vi "Read Connection Configuration.vi"(8 "error in (no error)":errorcluster, 11 "OPC UA configuration in":refnum<class "OPC UA Server configuration.lvclass">) -> (0 "error out":errorcluster, 2 "Connection Configuration":T2={"Client?"=FALSE, "Server Certificates"={"Relative Path?"=FALSE, "Certificate Paths"=[], "Certificate Names"=[]}, "Client Certificates"={"Relative Path?"=FALSE, "Certificate Paths"=[], "Certificate Names"=[]}, "Client Configuration"={"Server Endpoint URL"="", "Security Policy"={"Message Mode"=enum."None", "Security"=enum."Basic256"}, "Username/Password"={"Username"="", "Password"=""}}, "Server Configuration"={"Server Name"="", "TCP port (49580)"="49580", "Supported Security Policies"={"None"=TRUE, "Sign with Basic128Rsa125"=FALSE, "Sign and Encrypt with Basic128Rsa125"=FALSE, "Sign with Basic256"=FALSE, "Sign and Encrypt with Basic256"=FALSE}}}, 3 "OPC UA configuration out":refnum<class "OPC UA Server configuration.lvclass">)   [LabVIEW 2013, in "OPC UA Server configuration.lvclass"]
uses:
  OPC UA Server configuration.lvclass
  <vilib>/OPCUA/server/subVI/supported security policies.ctl
  OPC UA Server configuration.lvclass/OPC UA Server configuration.ctl
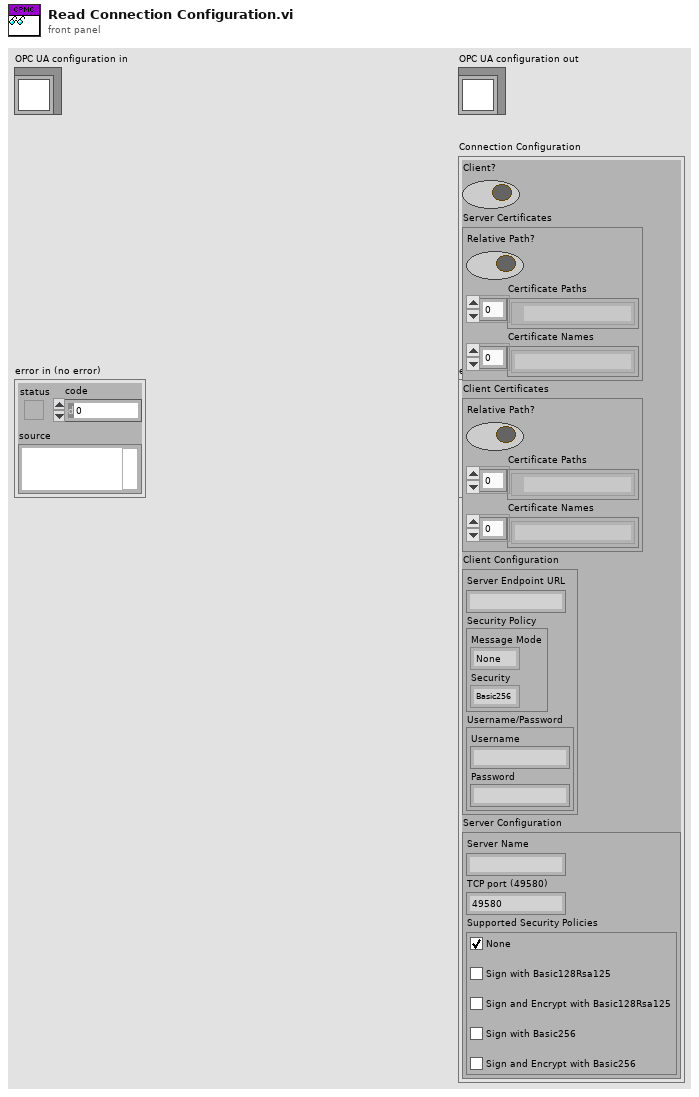
[diagram p1: front panel]
types:
  T1 = typedef "supported security policies.ctl" = cluster{"None":bool, "Sign with Basic128Rsa125":bool, "Sign and Encrypt with Basic128Rsa125":bool, "Sign with Basic256":bool, "Sign and Encrypt with Basic256":bool}
  T2 = cluster{"Client?":bool, "Server Certificates":cluster{"Relative Path?":bool, "Certificate Paths":path[], "Certificate Names":string[]}, "Client Certificates":cluster{"Relative Path?":bool, "Certificate Paths":path[], "Certificate Names":string[]}, "Client Configuration":cluster{"Server Endpoint URL":string, "Security Policy":cluster{"Message Mode":enum16{"None", "Sign", "Sign and Encrypt"}, "Security":enum16{"Basic256", "Basic128Rsa15"}}, "Username/Password":cluster{"Username":string, "Password":string}}, "Server Configuration":cluster{"Server Name":string, "TCP port (49580)":string, "Supported Security Policies":T1}}
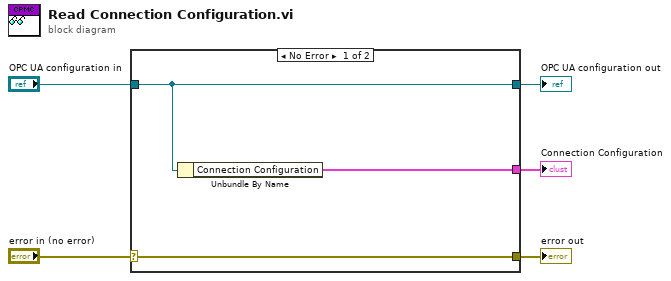
[diagram p0: block diagram]
diagram:
  n1 = case shown="No Error" "error in (no error)" {
    selector: "error in (no error)" -> [w8 w9]
    tunnel: [w8 w9] -> w4
    tunnel: [w7 w10] -> w2
    tunnel: "OPC UA configuration in" -> [w7 w10]
    tunnel: [w6 _] -> w1
    frame No Error {
      n2 = Unbundle By Name(w7) -> ("Connection Configuration"=w6:T2)
    }
    frame Error {
    }
  }
  "error out" <- w4
  "OPC UA configuration out" <- w2
  "Connection Configuration" <- w1
